vi "Send TCP-IP Cmd and Get Ackn 3.vi"(0 "TCP/IP ID In":refnum<k5>, 7 "Cmd Packet":string, 11 "error in (no error)":errorcluster) -> (2 "TCP/IP ID Out":refnum<k5>, 3 "Read String":string, 4 "Packet Length":u32, 6 "Packet ID":u8, 8 "Camera ID":u8, 10 "Accepted Flag":bool, 15 "error out":errorcluster)   [LabVIEW 2015]
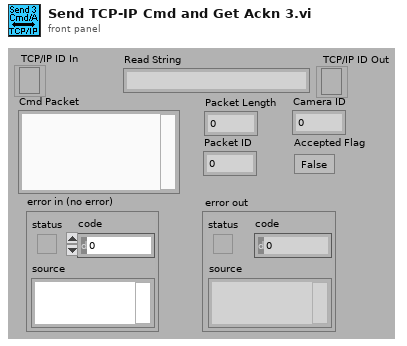
[diagram p1: front panel]
types:
  T1 = cluster{"Packet Length":u32, "Packet ID":u8, "Camera ID":u8, "Accepted Flag":u16}
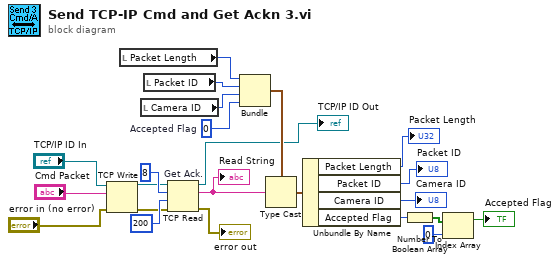
[diagram p0: block diagram]
diagram:
  w16 = u16 0  # Accepted Flag
  n1 = TCP Write(connection ID="TCP/IP ID In", data in="Cmd Packet", error in (no error)="error in (no error)") -> (connection ID out=w19:refnum<k5>, error out=w21:errorcluster)  [unwired: 1 in, 1 out]
  n2 = local read "Packet Length"() -> (w5:u32)
  n3 = local read "Camera ID"() -> (w17:u8)
  n4 = local read "Packet ID"() -> (w4:u8)
  n5 = TCP Read "Get Ack."(connection ID=w19, bytes to read=8, error in (no error)=w21, 9:200 ("timeout ms (25000)")) -> (connection ID out=→"TCP/IP ID Out":refnum<k5>, data out=w14:string, error out=→"error out":errorcluster)  [unwired: 1 in]
  "Read String" <- w14
  n6 = Bundle("Packet Length"=w5, "Packet ID"=w4, "Camera ID"=w17, "Accepted Flag"=w16) -> (w15:T1)  [unwired: 1 in]
  n7 = Type Cast(type=w15, x=w14) -> (*(type *) &x=w13:T1)
  n8 = Unbundle By Name(w13) -> ("Packet Length"=→"Packet Length":u32, "Packet ID"=→"Packet ID":u8, "Camera ID"=→"Camera ID":u8, "Accepted Flag"=w11:u16)
  n9 = Number To Boolean Array(number=w11) -> (Boolean array=w10:bool[])
  n10 = Index Array(array=w10, index=0 ("Index")) -> (element=→"Accepted Flag":bool)
